vi "Get Section.vi"(8 "sections":string[](array[string]), 11 "info data":string) -> (0 "sections out":string[](array[string]), 1 "exist":bool, 3 "section part":string)   [LabVIEW 2020, in "infolib.lvlib"]
doc: "Finds section structure and return its content. If not found, exist is false. If no section structure set, returns whole info data and exist is true."
uses:
  infolib.lvlib
  <vilib>/Utility/error.llb/whitespace.ctl
  <vilib>/regexp/Match Regular Expression.xnode
panel:
  # "testing string: (put \"1\" and \"2\" into section names)"
  # "blfdablad\n#startsection:: 1\njfkdla\n#startsection:: 2\ngroup2group2\n\t  \t#endsection:: 2\njdfkls\n#endsection:: 1\njfdklajfkdl"
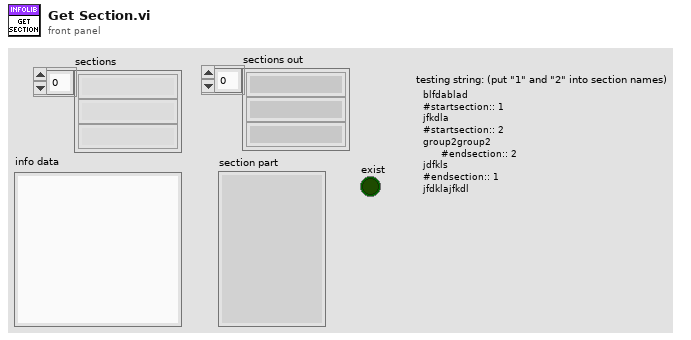
[diagram p1: front panel]
types:
  T1 = typedef "whitespace.ctl" = u16
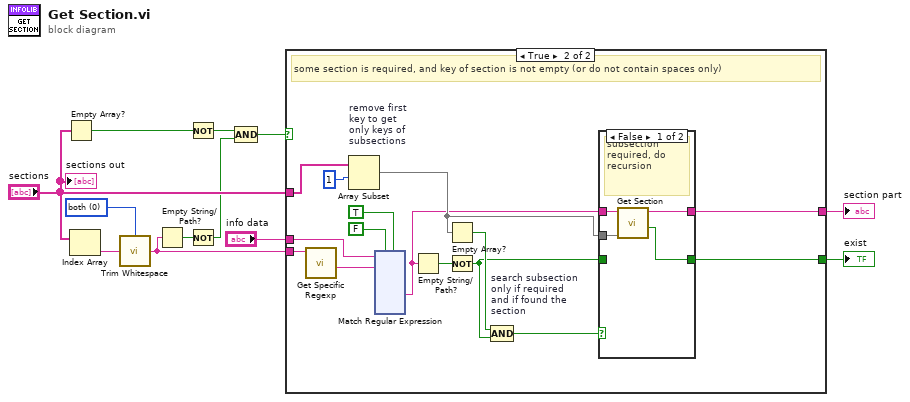
[diagram p0: block diagram]
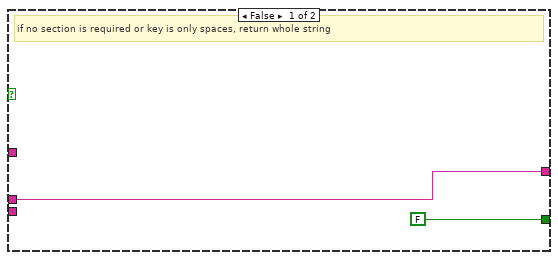
[diagram p2: hidden frame]
diagram:
  w7 = T1 0 items=["both", "start of string", "end of string"] ("location (both)")
  n1 = Empty Array?(array="sections") -> (empty?=w4:bool)
  n2 = Index Array(array="sections") -> (element=w8:string)  [unwired: 1 in]
  n3 = call <vilib>:"Trim Whitespace.vi"("string"=w8, "location (both)"=w7) -> ("trimmed string"=w5:string)
  n4 = Empty String/Path?(string/path=w5) -> (empty?=w2:bool)
  n5 = Not(x=w4) -> (.not. x?=w3:bool)
  n6 = Not(x=w2) -> (.not. x?=w1:bool)
  n7 = Compound Arithmetic op=AND(w3, w1) -> (w6:bool)
  n8 = case shown="True" w6 {
    tunnel: "sections" -> [_ w27]
    tunnel: "info data" -> [w13 w29]
    tunnel: [w13 w25] -> w10
    tunnel: [FALSE ("exist") w24] -> w9
    tunnel: w5 -> [_ w17]
    frame False {
      # "if no section is required or key is only spaces, return whole string"
    }
    frame True {
      # "some section is required, and key of section is not empty (or do not contain spaces only)"
      n9 = call "Get Specific Regexp.vi"("key of line, of matrix, of section ('')"=w17) -> ("Section"=w21:string)  [unwired: 7 in, 3 out]
      n10 = Array Subset "remove first\nkey to get\nonly keys of\nsubsections"(array=w27, index=1) -> (w26:string[])  [unwired: 1 in]
      n11 = xnode "Match Regular Expression"("input string"=w29, "regular expression"=w21, "ignore case? (F)"=FALSE, "multiline? (F)"=TRUE) -> ("submatch 1"=w15:string)  [unwired: 2 in, 7 out]
      n12 = Empty String/Path?(string/path=w15) -> (empty?=w20:bool)
      n13 = Empty Array?(array=w26) -> (empty?=w19:bool)
      n14 = Not(x=w20) -> (.not. x?=w16:bool)
      n15 = Compound Arithmetic op=AND "search subsection\nonly if required\nand if found the\nsection"(w19, w16) -> (w18:bool)
      n16 = case shown="False" w18 {
        tunnel: w15 -> [w151 w153]
        tunnel: [w150 w153] -> w25
        tunnel: w26 -> [w149 _]
        tunnel: [w148 w152] -> w24
        tunnel: w16 -> [_ w152]
        frame False {
          # "subsection\nrequired, do\nrecursion"
          n17 = call "Get Section.vi"("sections"=w149, "info data"=w151) -> ("exist"=w148:bool, "section part"=w150:string)  [unwired: 7 in, 1 out]
        }
        frame True {
          # "subsection not\nrequired"
        }
      }
    }
  }
  "exist" <- w9
  "section part" <- w10
  "sections out" <- "sections"
